vi "定时控制后台任务.vi"   [LabVIEW 2016]
uses:
  Holding Var.vi
  random number/random number.lvlib
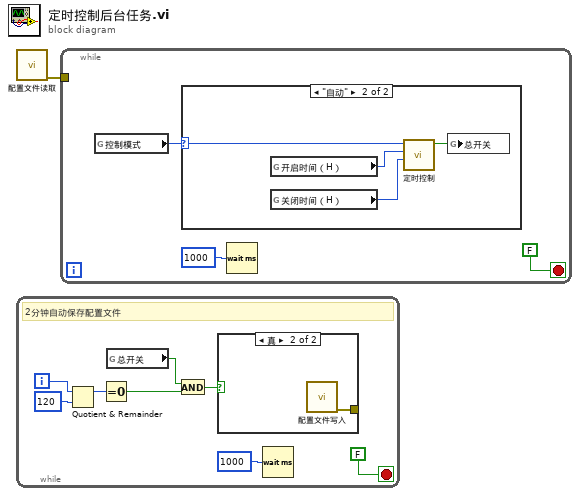
[diagram p0: block diagram]
diagram:
  n1 = call "配置文件读取.vi"() -> ("error out"=w1:errorcluster)  [unwired: 11 in]
  n2 = while {
    i -> [w7]
    stop <- FALSE stop-if-true
    # "2分钟自动保存配置文件"
    n3 = Quotient & Remainder(x=w7, y=120) -> (x-y*floor(x/y)=w5:i32)  [unwired: 1 out]
    n4 = Equal To 0?(x=w5) -> (x = 0?=w4:bool)
    n5 = global read "Holding Var.vi" "总开关"() -> (w2:bool)
    n6 = And(x=w2, y=w4) -> (x .and. y?=w3:bool)
    n7 = case shown="真" w3 {
      tunnel: [_ w10] -> _
      frame False {
      }
      frame True {
        n8 = call "配置文件写入.vi"() -> ("错误输出"=w10:errorcluster)  [unwired: 11 in]
      }
    }
    n9 = Wait (ms)(milliseconds to wait=u32 1000 ("等待时间（毫秒）")) -> ()  [unwired: 1 out]
  }
  n10 = while {
    tunnel: w1 -> [_]
    stop <- FALSE stop-if-true
    n11 = global read "Holding Var.vi" "控制模式"() -> (w13:enum16{"手动", "自动"})
    n12 = case shown="\"自动\"" w13 {
      selector: w13 -> [_ w14]
      frame "手动", Default {
      }
      frame "自动" {
        n13 = global read "Holding Var.vi" "开启时间（H）"() -> (w17:u16)
        n14 = global read "Holding Var.vi" "关闭时间（H）"() -> (w16:u16)
        n15 = call "定时控制.vi"("关闭时间（H）"=w16, "开启时间（H）"=w17, "控制模式"=w14) -> ("布尔"=w15:bool)  [unwired: 8 in]
        n16 = global write "Holding Var.vi" "总开关"(w15) -> ()
      }
    }
    n17 = Wait (ms)(milliseconds to wait=u32 1000 ("等待时间（毫秒）")) -> ()  [unwired: 1 out]
  }
